vi "Append Watermark polymorphic.vi"   [LabVIEW 2019]
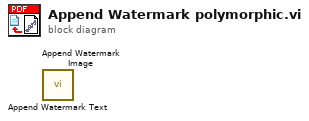
[diagram p0: block diagram]
diagram:
  n1 = call <userlib>:"Append Watermark Text.vi"() -> ()  [unwired: 14 in, 2 out]
  n2 = call <userlib>:"Append Watermark Image.vi"() -> ()  [unwired: 14 in, 2 out]
